vi "simple_loadcell.vi"() -> ()   [LabVIEW 2013]
uses:
  <vilib>/DAQmx/read.llb/DAQmx Read.vi
  <vilib>/DAQmx/read.llb/DAQmx Read (Analog Wfm 1Chan NSamp).vi
  <vilib>/Analysis/baseanly.llb/Mean (DBL).vi
  <vilib>/DAQmx/create/channels.llb/DAQmx Create Channel (AI-Voltage-Basic).vi
  <vilib>/DAQmx/configure/timing.llb/DAQmx Timing (Sample Clock).vi
  <vilib>/DAQmx/miscellaneous.llb/DAQmx Fill In Error Info.vi
  <vilib>/Analysis/NI_AALBase.lvlib
  <resource>/objmgr/daqmx.rc
panel:
  out "mean":dbl caption="평균" format="%.6f"
  out "g":dbl caption="평균" format="%.6f"
  in  "null":bool
  out "웨이브폼 차트":dbl(graph)
  out "data":waveform(dbl)(graph) caption="데이터"
  in  "stop":bool caption="정지"
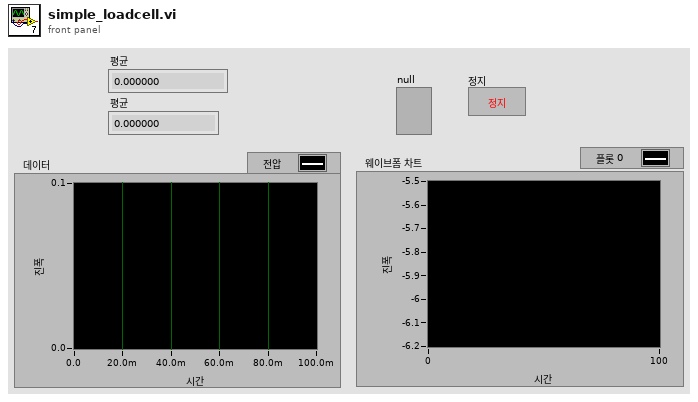
[diagram p1: front panel]
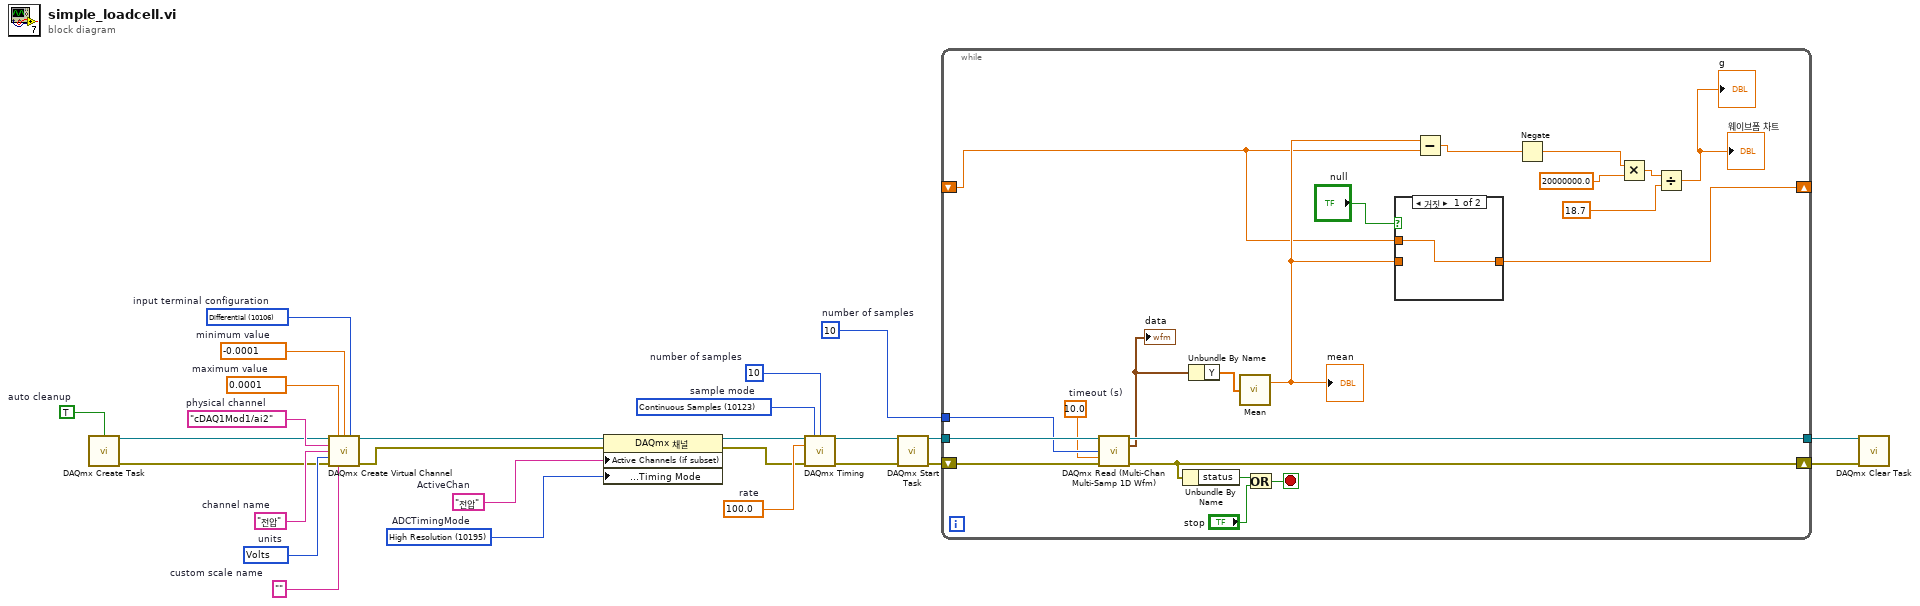
[diagram p0: block diagram]
diagram:
  w21 = 10123 items=["Finite Samples"=10178, "Continuous Samples"=10123, "Hardware Timed Single Point"=12522]  # sample mode
  w20 = 10  # number of samples
  w19 = 100.0  # rate
  w16 = 10195 items=["High Resolution"=10195, "High Speed"=14712, "Best 50 Hz Rejection"=14713, "Best 60 Hz Rejection"=14714]  # ADCTimingMode
  w14 = "전압"  # ActiveChan
  w13 = 10106 items=["default"=-1, "RSE"=10083, "NRSE"=10078, "Differential"=10106, "Pseudodifferential"=12529]  # input terminal configuration
  w12 = 10348 items=["Volts"=10348, "From Custom Scale"=10065]  # units
  w11 = "전압"  # channel name
  w9 = ""  # custom scale name
  w8 = -0.0001  # minimum value
  w7 = 0.0001  # maximum value
  w6 = "cDAQ1Mod1/ai2"  # physical channel
  w4 = TRUE  # auto cleanup
  w24 = 10  # number of samples
  n1 = call <vilib>:"DAQmx Create Task.vi"("auto cleanup"=w4) -> ("task out"=w5:refnum<k21>, "error out"=w3:errorcluster)  [unwired: 13 in]
  n2 = call-poly <vilib>:"DAQmx Create Virtual Channel.vi"("task in"=w5, "maximum value"=w7, "minimum value"=w8, "input terminal configuration"=w13, "physical channels"=w6, "name to assign"=w11, "units"=w12, "error in"=w3, "custom scale name"=w9) -> ("task out"=w17:refnum<k21>, "error out"=w10:errorcluster)  [unwired: 5 in]
  n3 = property class="DAQmx 채널"(reference=w17, error in=w10, "Active Channels (if subset)"=w14, "Analog Input:General Properties:Digitizer/ADC:Timing Mode"=w16) -> (reference out=w18:refnum<k21>, error out=w15:errorcluster)
  n4 = call-poly <vilib>:"DAQmx Timing.vi"("task/channels in"=w18, "sample mode"=w21, "samples per channel"=w20, "rate"=w19, "error in"=w15) -> ("task out"=w1:refnum<k21>, "error out"=w2:errorcluster)  [unwired: 9 in]
  n5 = call <vilib>:"DAQmx Start Task.vi"("task/channels in"=w1, "error in"=w2) -> ("task out"=w26:refnum<k21>, "error out"=w25:errorcluster)  [unwired: 12 in]
  n6 = while "While 루프" {
    tunnel: w26 -> [w47]
    tunnel: w24 -> [w44]
    tunnel: [w45] -> w22
    shift-right: [w42] -> w23
    shift-left: w25 -> [w46]
    shift-right: [w34] -> _
    shift-left: _ -> [w33]
    stop <- w41 stop-if-true
    w39 = 10.0  # timeout (s)
    n7 = call-poly "DAQmx Read (Multi-Chan Multi-Samp 1D Wfm).vi"("task/channels in"=w47, "number of samples per channel"=w44, "timeout"=w39, "error in"=w46) -> ("task out"=w45:refnum<k21>, "data"=w37:waveform(dbl), "error out"=w42:errorcluster)  [unwired: 9 in]
    "data" <- w37
    n8 = Unbundle By Name(w42) -> ("status"=w43:bool)
    n9 = Unbundle By Name(w37) -> ("Y"=w38:dbl[])
    n10 = call-poly <vilib>:"Mean.vi"("X"=w38) -> ("mean"=w35:dbl)  [unwired: 1 out]
    "mean" <- w35
    n11 = Or(x=w43, y="stop") -> (x .or. y?=w41:bool)
    n12 = case shown="거짓" "null" {
      tunnel: w35 -> [_ w49]
      tunnel: [w48 w49] -> w34
      tunnel: w33 -> [w48 _]
      frame False {
      }
      frame True {
      }
    }
    n13 = Subtract(x=w35, y=w33) -> (x-y=w30:dbl)
    n14 = Negate(x=w30) -> (-x=w29:dbl)
    n15 = Multiply(x=w29, y=20000000.0) -> (x*y=w31:dbl)
    n16 = Divide(x=w31, y=18.7) -> (x/y=→"웨이브폼 차트" →"g":dbl)
  }
  n17 = call <vilib>:"DAQmx Clear Task.vi"("task in"=w22, "error in"=w23) -> ()  [unwired: 13 in, 1 out]
